vi "Project 7 - Johnson.vi"() -> ()   [LabVIEW 2019]
uses:
  <vilib>/Instr/_visa.llb/VISA Configure Serial Port (Instr).vi
panel:
  in  "Freq":string
  in  "Ohms":string
  in  "Amps":string
  in  "Volts":string
  in  "Tab Control":enum32{"Measurements", "Settings"}(tab)
  in  "Func1":T1(ring)=enum."VDC"
  out "Measure2":dbl
  in  "Func2":T1(ring)=enum."VDC"
  in  "Read":bool
  out "Measure1":dbl
  in  "stop":bool
  in  "Ch Mode":bool
  in  "VISA resource name":refnum<visa-resource-name>="COM5"
  out "error out":errorcluster
  # "CH 1"
  # "CH 2"
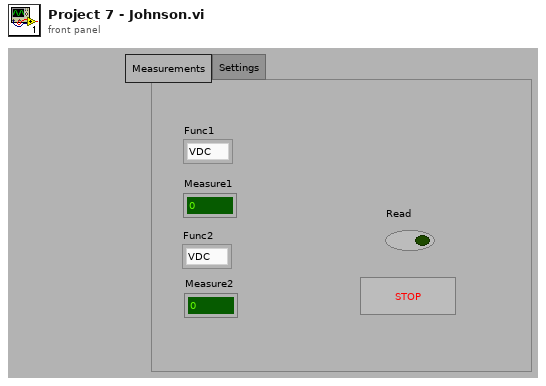
[diagram p1: front panel]
types:
  T1 = enum16{"AAC", "ADC", "CONT", "DIODE", "FREQ", "OHMS", "VAC", "VDC"}
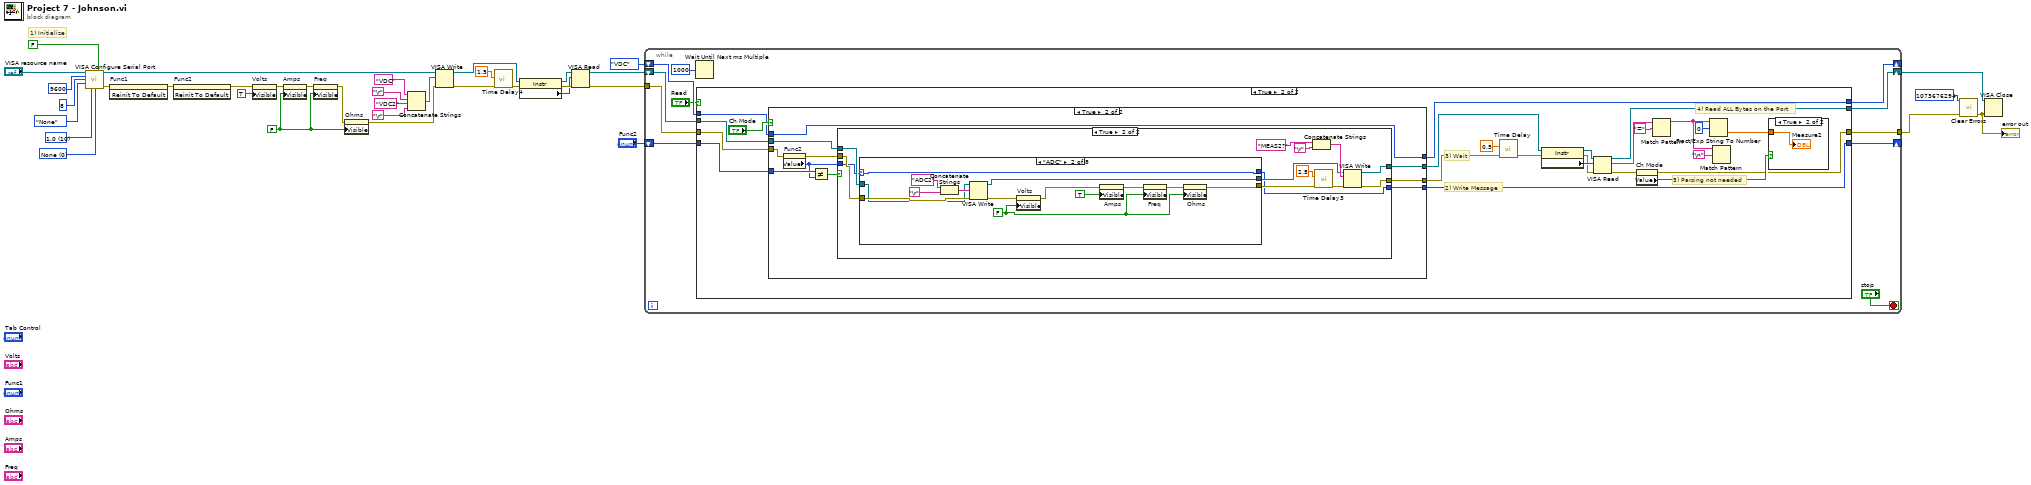
[diagram p0: block diagram]
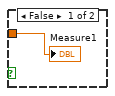
[diagram p3: hidden frame]
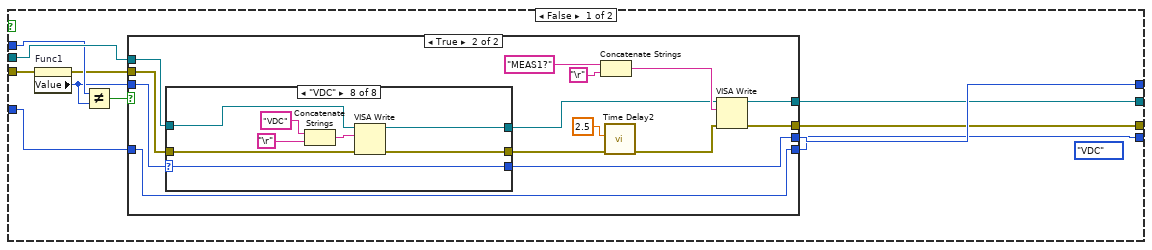
[diagram p4: hidden frame]
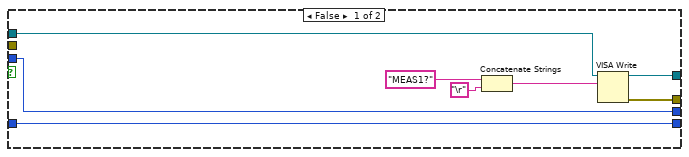
[diagram p5: hidden frame]
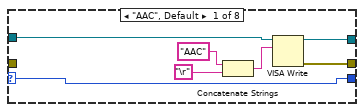
[diagram p6: hidden frame]
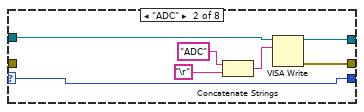
[diagram p7: hidden frame]
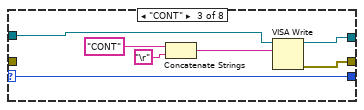
[diagram p8: hidden frame]
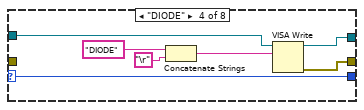
[diagram p9: hidden frame]
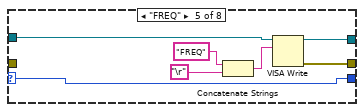
[diagram p10: hidden frame]
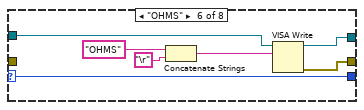
[diagram p11: hidden frame]
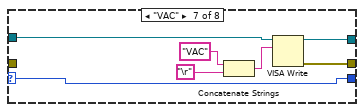
[diagram p12: hidden frame]
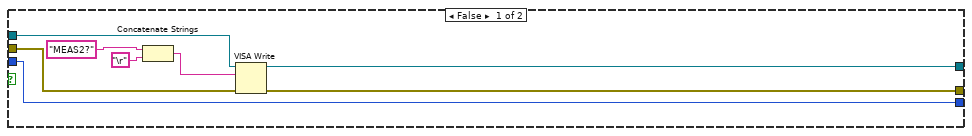
[diagram p13: hidden frame]
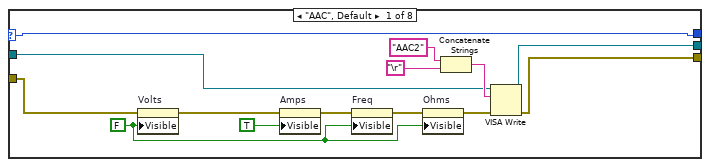
[diagram p14: hidden frame]
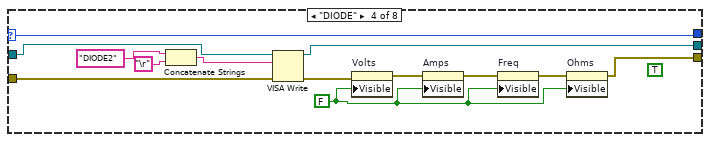
[diagram p16: hidden frame]
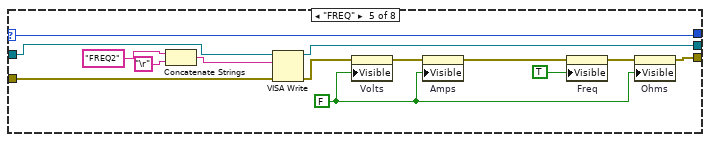
[diagram p17: hidden frame]
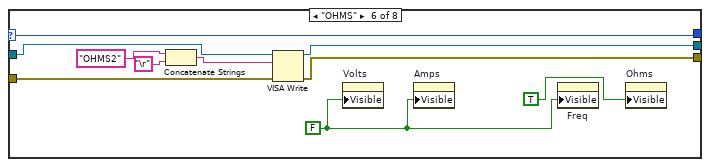
[diagram p18: hidden frame]
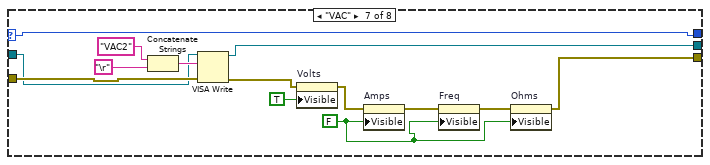
[diagram p19: hidden frame]
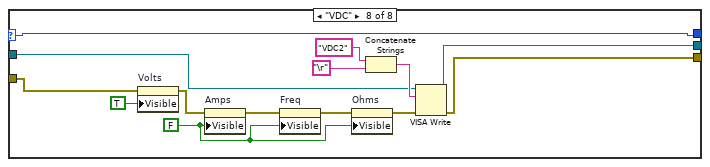
[diagram p20: hidden frame]
diagram:
  w8 = FALSE
  w29 = u16 0 items=["None", "XON/XOFF", "RTS/CTS", "XON/XOFF & RTS/CTS", "DTR/DSR", "XON/XOFF & DTR/DSR"] ("flow control (0:none)")
  w30 = u16 10 items=["1.0"=10, "1.5"=15, "2.0"=20] ("stop bits (10: 1 bit)")
  # "1) Initialize"
  n1 = call-poly "VISA Configure Serial Port"("VISA resource name"="VISA resource name", "Enable Termination\nChar (T)"=FALSE ("Enable Termination\nChar (T)"), "baud rate (9600)"=u32 9600, "data bits (8)"=u16 8, "parity (0:none)"=enum16{"None", "Odd", "Even", "Mark", "Space"}."None", "stop bits (10: 1 bit)"=w30, "flow control (0:none)"=w29) -> ("VISA resource name out"=w22:refnum<visa-resource-name>, "error out"=w17:errorcluster)  [unwired: 1 in, 6 out]
  n2 = invoke on="Func1" class="Enum (strict)" method="Reinit To Default"(error in=w17) -> (error out=w16:errorcluster)  [unwired: 2 in, 2 out]
  n3 = invoke on="Func2" class="Enum (strict)" method="Reinit To Default"(error in=w16) -> (error out=w6:errorcluster)  [unwired: 2 in, 2 out]
  n4 = property on="Volts" class="Str"(error in=w6, "Visible"=TRUE) -> (error out=w5:errorcluster)  [unwired: 1 in, 1 out]
  n5 = property on="Amps" class="Str"(error in=w5, "Visible"=w8) -> (error out=w4:errorcluster)  [unwired: 1 in, 1 out]
  n6 = property on="Freq" class="Str"(error in=w4, "Visible"=w8) -> (error out=w3:errorcluster)  [unwired: 1 in, 1 out]
  n7 = property on="Ohms" class="Str"(error in=w3, "Visible"=w8) -> (error out=w2:errorcluster)  [unwired: 1 in, 1 out]
  n8 = Concatenate Strings("VDC" ("string"), "\r", "VDC2" ("string"), "\r") -> (w25:string)
  n9 = VISA Write(VISA resource name=w22, write buffer=w25, error in (no error)=w2) -> (VISA resource name out=w12:refnum<visa-resource-name>, error out=w19:errorcluster)  [unwired: 1 out]
  n10 = call "Time Delay4"("error in (no error)"=w19, "Delay Time (s)"=1.5) -> ("error out"=w10:errorcluster)  [unwired: 9 out]
  n11 = property on="Property Node" class="Instr"(reference=w12, error in=w10) -> (reference out=w14:refnum<visa-resource-name>, error out=w15:errorcluster, "Serial Settings:Number of Bytes at Serial Port"=w13:u32)
  n12 = VISA Read(VISA resource name=w14, byte count=w13, error in (no error)=w15) -> (VISA resource name out=w11:refnum<visa-resource-name>, error out=w9:errorcluster)  [unwired: 2 out]
  n13 = while {
    tunnel: w9 -> [w47]
    tunnel: [w44] -> w26
    shift-right: [w45] -> w36
    shift-left: w11 -> [w48]
    shift-right: [w41] -> _
    shift-left: T1."VDC" ("Func1") -> [w42]
    shift-right: [w39] -> _
    shift-left: "Func2" -> [w40]
    stop <- "stop" stop-if-true
    n14 = Wait Until Next ms Multiple(millisecond multiple=u32 1000) -> ()  [unwired: 1 out]
    n15 = case shown="True" "Read" {
      tunnel: w48 -> [w52 w63]
      tunnel: w47 -> [w51 w59]
      tunnel: [w52 w76] -> w45
      tunnel: [w51 w53] -> w44
      tunnel: w42 -> [w50 w64]
      tunnel: [w50 w60] -> w41
      tunnel: w40 -> [w49 w58]
      tunnel: [w49 w57] -> w39
      frame False {
      }
      frame True {
        # "5) Parsing not needed"
        # "3) Wait"
        # "2) Write Message"
        # "4) Read ALL Bytes on the Port"
        n16 = case shown="True" "Ch Mode" {
          tunnel: w64 -> [w87 w169]
          tunnel: w59 -> [w80 w175]
          tunnel: w63 -> [w89 w178]
          tunnel: [w84 w173] -> w62
          tunnel: [w85 w174] -> w61
          tunnel: [w88 w169] -> w60
          tunnel: w58 -> [w83 w172]
          tunnel: [w82 w171] -> w57
          frame False {
            (unwired) T1."VDC" ("Func1")
            n17 = property on="Func1" class="Enum (strict)"(error in=w80) -> (error out=w79:errorcluster, "Value"=w81:T1)  [unwired: 1 in, 1 out]
            n18 = Not Equal?(x=w87, y=w81) -> (x != y?=w86:bool)
            n19 = case shown="True" w86 {
              tunnel: w89 -> [w92 w111]
              tunnel: [w93 w101] -> w84
              tunnel: [w94 w99] -> w85
              tunnel: [w90 w110] -> w88
              tunnel: w83 -> [w91 w107]
              tunnel: [w91 w107] -> w82
              tunnel: w81 -> [w90 w106]
              tunnel: w79 -> [_ w98]
              frame False {
                n20 = Concatenate Strings("MEAS1?" ("string"), "\r") -> (w97:string)
                n21 = VISA Write(VISA resource name=w92, write buffer=w97) -> (VISA resource name out=w93:refnum<visa-resource-name>, error out=w94:errorcluster)  [unwired: 1 in, 1 out]
              }
              frame True {
                n22 = case shown="\"VDC\"" w106 {
                  selector: w106 -> [w112 w119 w126 w133 w140 w147 w154 w162]
                  tunnel: [w115 w122 w129 w136 w143 w150 w157 w165] -> w102
                  tunnel: w111 -> [w114 w121 w128 w135 w142 w149 w156 w164]
                  tunnel: [w113 w120 w127 w134 w141 w148 w155 w163] -> w108
                  tunnel: [w112 w119 w126 w133 w140 w147 w154 w162] -> w110
                  tunnel: w98 -> [_ _ _ _ _ _ _ w161]
                  frame "AAC", Default {
                    n23 = Concatenate Strings("AAC" ("string"), "\r") -> (w118:string)
                    n24 = VISA Write(VISA resource name=w114, write buffer=w118) -> (VISA resource name out=w115:refnum<visa-resource-name>, error out=w113:errorcluster)  [unwired: 1 in, 1 out]
                  }
                  frame "ADC" {
                    n25 = Concatenate Strings("ADC" ("string"), "\r") -> (w125:string)
                    n26 = VISA Write(VISA resource name=w121, write buffer=w125) -> (VISA resource name out=w122:refnum<visa-resource-name>, error out=w120:errorcluster)  [unwired: 1 in, 1 out]
                  }
                  frame "CONT" {
                    n27 = Concatenate Strings("CONT" ("string"), "\r") -> (w132:string)
                    n28 = VISA Write(VISA resource name=w128, write buffer=w132) -> (VISA resource name out=w129:refnum<visa-resource-name>, error out=w127:errorcluster)  [unwired: 1 in, 1 out]
                  }
                  frame "DIODE" {
                    n29 = Concatenate Strings("DIODE" ("string"), "\r") -> (w139:string)
                    n30 = VISA Write(VISA resource name=w135, write buffer=w139) -> (VISA resource name out=w136:refnum<visa-resource-name>, error out=w134:errorcluster)  [unwired: 1 in, 1 out]
                  }
                  frame "FREQ" {
                    n31 = Concatenate Strings("FREQ" ("string"), "\r") -> (w146:string)
                    n32 = VISA Write(VISA resource name=w142, write buffer=w146) -> (VISA resource name out=w143:refnum<visa-resource-name>, error out=w141:errorcluster)  [unwired: 1 in, 1 out]
                  }
                  frame "OHMS" {
                    n33 = Concatenate Strings("OHMS" ("string"), "\r") -> (w153:string)
                    n34 = VISA Write(VISA resource name=w149, write buffer=w153) -> (VISA resource name out=w150:refnum<visa-resource-name>, error out=w148:errorcluster)  [unwired: 1 in, 1 out]
                  }
                  frame "VAC" {
                    n35 = Concatenate Strings("VAC" ("string"), "\r") -> (w160:string)
                    n36 = VISA Write(VISA resource name=w156, write buffer=w160) -> (VISA resource name out=w157:refnum<visa-resource-name>, error out=w155:errorcluster)  [unwired: 1 in, 1 out]
                  }
                  frame "VDC" {
                    n37 = Concatenate Strings("VDC" ("string"), "\r") -> (w168:string)
                    n38 = VISA Write(VISA resource name=w164, write buffer=w168, error in (no error)=w161) -> (VISA resource name out=w165:refnum<visa-resource-name>, error out=w163:errorcluster)  [unwired: 1 out]
                  }
                }
                n39 = Concatenate Strings("MEAS1?" ("string"), "\r") -> (w105:string)
                n40 = call "Time Delay2"("error in (no error)"=w108, "Delay Time (s)"=2.5) -> ("error out"=w100:errorcluster)  [unwired: 9 out]
                n41 = VISA Write(VISA resource name=w102, write buffer=w105, error in (no error)=w100) -> (VISA resource name out=w101:refnum<visa-resource-name>, error out=w99:errorcluster)  [unwired: 1 out]
              }
            }
          }
          frame True {
            n42 = property on="Func2" class="Enum (strict)"(error in=w175) -> (error out=w176:errorcluster, "Value"=w170:T1)  [unwired: 1 in, 1 out]
            n43 = Not Equal?(x=w172, y=w170) -> (x != y?=w177:bool)
            n44 = case shown="True" w177 {
              tunnel: w176 -> [w180 w199]
              tunnel: w178 -> [w181 w198]
              tunnel: [w182 w191] -> w173
              tunnel: [w183 w190] -> w174
              tunnel: [w179 w187] -> w171
              tunnel: w170 -> [w179 w188]
              frame False {
                n45 = Concatenate Strings("MEAS2?" ("string"), "\r") -> (w186:string)
                n46 = VISA Write(VISA resource name=w181, write buffer=w186, error in (no error)=w180) -> (VISA resource name out=w182:refnum<visa-resource-name>, error out=w183:errorcluster)  [unwired: 1 out]
              }
              frame True {
                n47 = case shown="\"ADC\"" w188 {
                  selector: w188 -> [w207 w221 w228 w237 w251 w260 w275 w289]
                  tunnel: w199 -> [w203 w224 w230 w240 w254 w264 w278 w286]
                  tunnel: [w210 w223 w229 w239 w253 w263 w277 w292] -> w192
                  tunnel: w198 -> [w209 w222 w229 w238 w252 w262 w276 w291]
                  tunnel: [w208 w215 w230 w232 w245 w261 w269 w290] -> w196
                  tunnel: [w207 w221 w228 w237 w251 w260 w275 w289] -> w187
                  frame "AAC", Default {
                    w200 = FALSE
                    n48 = property on="Volts" class="Str"(error in=w203, "Visible"=w200) -> (error out=w206:errorcluster)  [unwired: 1 in, 1 out]
                    n49 = property on="Amps" class="Str"(error in=w206, "Visible"=TRUE) -> (error out=w205:errorcluster)  [unwired: 1 in, 1 out]
                    n50 = property on="Freq" class="Str"(error in=w205, "Visible"=w200) -> (error out=w204:errorcluster)  [unwired: 1 in, 1 out]
                    n51 = property on="Ohms" class="Str"(error in=w204, "Visible"=w200) -> (error out=w202:errorcluster)  [unwired: 1 in, 1 out]
                    n52 = Concatenate Strings("AAC2" ("string"), "\r") -> (w213:string)
                    n53 = VISA Write(VISA resource name=w209, write buffer=w213, error in (no error)=w202) -> (VISA resource name out=w210:refnum<visa-resource-name>, error out=w208:errorcluster)  [unwired: 1 out]
                  }
                  frame "ADC" {
                    w214 = FALSE
                    n54 = Concatenate Strings("ADC2" ("string"), "\r") -> (w227:string)
                    n55 = VISA Write(VISA resource name=w222, write buffer=w227, error in (no error)=w224) -> (VISA resource name out=w223:refnum<visa-resource-name>, error out=w216:errorcluster)  [unwired: 1 out]
                    n56 = property on="Volts" class="Str"(error in=w216, "Visible"=w214) -> (error out=w220:errorcluster)  [unwired: 1 in, 1 out]
                    n57 = property on="Amps" class="Str"(error in=w220, "Visible"=TRUE) -> (error out=w219:errorcluster)  [unwired: 1 in, 1 out]
                    n58 = property on="Freq" class="Str"(error in=w219, "Visible"=w214) -> (error out=w218:errorcluster)  [unwired: 1 in, 1 out]
                    n59 = property on="Ohms" class="Str"(error in=w218, "Visible"=w214) -> (error out=w215:errorcluster)  [unwired: 1 in, 1 out]
                  }
                  frame "CONT" {
                  }
                  frame "DIODE" {
                    (unwired) TRUE ("Visible")
                    w231 = FALSE
                    n60 = Concatenate Strings("DIODE2" ("string"), "\r") -> (w243:string)
                    n61 = VISA Write(VISA resource name=w238, write buffer=w243, error in (no error)=w240) -> (VISA resource name out=w239:refnum<visa-resource-name>, error out=w233:errorcluster)  [unwired: 1 out]
                    n62 = property on="Volts" class="Str"(error in=w233, "Visible"=w231) -> (error out=w236:errorcluster)  [unwired: 1 in, 1 out]
                    n63 = property on="Amps" class="Str"(error in=w236, "Visible"=w231) -> (error out=w235:errorcluster)  [unwired: 1 in, 1 out]
                    n64 = property on="Freq" class="Str"(error in=w235, "Visible"=w231) -> (error out=w234:errorcluster)  [unwired: 1 in, 1 out]
                    n65 = property on="Ohms" class="Str"(error in=w234, "Visible"=w231) -> (error out=w232:errorcluster)  [unwired: 1 in, 1 out]
                  }
                  frame "FREQ" {
                    w247 = FALSE
                    n66 = Concatenate Strings("FREQ2" ("string"), "\r") -> (w257:string)
                    n67 = VISA Write(VISA resource name=w252, write buffer=w257, error in (no error)=w254) -> (VISA resource name out=w253:refnum<visa-resource-name>, error out=w246:errorcluster)  [unwired: 1 out]
                    n68 = property on="Volts" class="Str"(error in=w246, "Visible"=w247) -> (error out=w250:errorcluster)  [unwired: 1 in, 1 out]
                    n69 = property on="Amps" class="Str"(error in=w250, "Visible"=w247) -> (error out=w249:errorcluster)  [unwired: 1 in, 1 out]
                    n70 = property on="Freq" class="Str"(error in=w249, "Visible"=TRUE) -> (error out=w248:errorcluster)  [unwired: 1 in, 1 out]
                    n71 = property on="Ohms" class="Str"(error in=w248, "Visible"=w247) -> (error out=w245:errorcluster)  [unwired: 1 in, 1 out]
                  }
                  frame "OHMS" {
                    w259 = FALSE
                    n72 = Concatenate Strings("OHMS2" ("string"), "\r") -> (w267:string)
                    n73 = VISA Write(VISA resource name=w262, write buffer=w267, error in (no error)=w264) -> (VISA resource name out=w263:refnum<visa-resource-name>, error out=w261:errorcluster)  [unwired: 1 out]
                    n74 = property on="Volts" class="Str"("Visible"=w259) -> ()  [unwired: 2 in, 2 out]
                    n75 = property on="Amps" class="Str"("Visible"=w259) -> ()  [unwired: 2 in, 2 out]
                    n76 = property on="Freq" class="Str"("Visible"=w259) -> ()  [unwired: 2 in, 2 out]
                    n77 = property on="Ohms" class="Str"("Visible"=TRUE) -> ()  [unwired: 2 in, 2 out]
                  }
                  frame "VAC" {
                    w268 = FALSE
                    n78 = Concatenate Strings("VAC2" ("string"), "\r") -> (w281:string)
                    n79 = VISA Write(VISA resource name=w276, write buffer=w281, error in (no error)=w278) -> (VISA resource name out=w277:refnum<visa-resource-name>, error out=w271:errorcluster)  [unwired: 1 out]
                    n80 = property on="Volts" class="Str"(error in=w271, "Visible"=TRUE) -> (error out=w270:errorcluster)  [unwired: 1 in, 1 out]
                    n81 = property on="Amps" class="Str"(error in=w270, "Visible"=w268) -> (error out=w274:errorcluster)  [unwired: 1 in, 1 out]
                    n82 = property on="Freq" class="Str"(error in=w274, "Visible"=w268) -> (error out=w273:errorcluster)  [unwired: 1 in, 1 out]
                    n83 = property on="Ohms" class="Str"(error in=w273, "Visible"=w268) -> (error out=w269:errorcluster)  [unwired: 1 in, 1 out]
                  }
                  frame "VDC" {
                    w288 = FALSE
                    n84 = property on="Volts" class="Str"(error in=w286, "Visible"=TRUE) -> (error out=w285:errorcluster)  [unwired: 1 in, 1 out]
                    n85 = property on="Amps" class="Str"(error in=w285, "Visible"=w288) -> (error out=w284:errorcluster)  [unwired: 1 in, 1 out]
                    n86 = property on="Freq" class="Str"(error in=w284, "Visible"=w288) -> (error out=w283:errorcluster)  [unwired: 1 in, 1 out]
                    n87 = property on="Ohms" class="Str"(error in=w283, "Visible"=w288) -> (error out=w282:errorcluster)  [unwired: 1 in, 1 out]
                    n88 = Concatenate Strings("VDC2" ("string"), "\r") -> (w295:string)
                    n89 = VISA Write(VISA resource name=w291, write buffer=w295, error in (no error)=w282) -> (VISA resource name out=w292:refnum<visa-resource-name>, error out=w290:errorcluster)  [unwired: 1 out]
                  }
                }
                n90 = Concatenate Strings("MEAS2?" ("string"), "\r") -> (w195:string)
                n91 = call "Time Delay3"("error in (no error)"=w196, "Delay Time (s)"=2.5) -> ("error out"=w189:errorcluster)  [unwired: 9 out]
                n92 = VISA Write(VISA resource name=w192, write buffer=w195, error in (no error)=w189) -> (VISA resource name out=w191:refnum<visa-resource-name>, error out=w190:errorcluster)  [unwired: 1 out]
              }
            }
          }
        }
        n93 = call "Time Delay"("error in (no error)"=w61, "Delay Time (s)"=0.5) -> ("error out"=w72:errorcluster)  [unwired: 9 out]
        n94 = property on="Property Node" class="Instr"(reference=w62, error in=w72) -> (reference out=w74:refnum<visa-resource-name>, error out=w73:errorcluster, "Serial Settings:Number of Bytes at Serial Port"=w75:u32)
        n95 = VISA Read(VISA resource name=w74, byte count=w75, error in (no error)=w73) -> (VISA resource name out=w76:refnum<visa-resource-name>, read buffer=w70:string, error out=w54:errorcluster)  [unwired: 1 out]
        n96 = property on="Ch Mode" class="Bool (strict)"(error in=w54) -> (error out=w53:errorcluster, "Value"=w56:bool)  [unwired: 1 in, 1 out]
        n97 = Match Pattern(string=w70, regular expression="=") -> (before substring=w66:string)  [unwired: 1 in, 3 out]
        n98 = Fract/Exp String To Number(string=w66, offset=0) -> (number=w55:dbl)  [unwired: 2 in, 1 out]
        n99 = Match Pattern(string=w66, regular expression="\n") -> ()  [unwired: 1 in, 4 out]
        n100 = case shown="True" w56 {
          tunnel: w55 -> [w77 w78]
          frame False {
            "Measure1" <- w77
          }
          frame True {
            "Measure2" <- w78
          }
        }
      }
    }
  }
  n101 = call <vilib>:"Clear Errors.vi"("error in (no error)"=w26, "specific error code to clear (0: all)"=1073676294) -> ("error out"=w1:errorcluster)  [unwired: 4 in, 1 out]
  "error out" <- w1
  n102 = VISA Close(VISA resource name=w36, error in (no error)=w1) -> ()  [unwired: 1 out]
